vi "poly_control_signalling_write_caller_multi_2.vi"(6 "modes (Sgnl)":T1(array[ring]), 8 "error in (no error)":errorcluster, 9 "values":variant[](array[variant]), 10 "control names":string[](array[string]), 11 "name of caller in (your caller)":string) -> (0 "error out":errorcluster, 2 "control refs":refnum<vi>[](array[refnum]), 4 "found?":bool[](array[boolean]))   [LabVIEW 2015]
uses:
  poly_ref_tools_eco_plus.vi
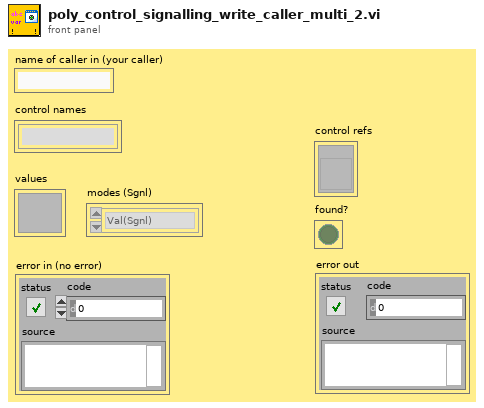
[diagram p1: front panel]
types:
  T1 = enum16{"Val", "Val(Sgnl)", "Val(Undo)", "Method"}[]
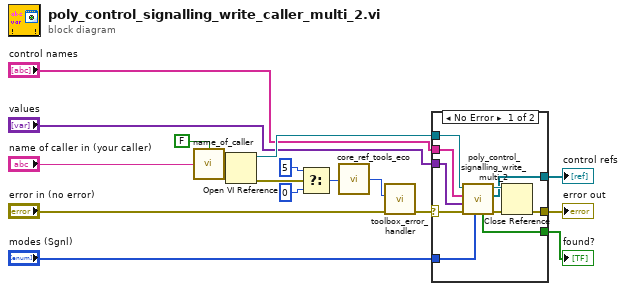
[diagram p0: block diagram]
diagram:
  n1 = call "name_of_caller.vi"("is in inlined vi? (F)"=FALSE, "name of caller in"="name of caller in (your caller)") -> ("name of caller out"=w16:string)  [unwired: 2 in]
  n2 = Open VI Reference(vi path=w16) -> (vi reference=w15:refnum<vi>, error out=w2:errorcluster)  [unwired: 5 in]
  n3 = Select(t=5, s=w2, f=0) -> (s? t:f=w5:i32)
  n4 = call-poly "core_ref_tools_eco.vi"("code (w/out eco)"=w5) -> ("code (+ eco)"=w4:i32)  [unwired: 4 in]
  n5 = call "toolbox_error_handler.vi"("error in (no error)"="error in (no error)", "code (0 = no error)"=w4) -> ("error out"=w1:errorcluster)  [unwired: 8 in, 1 out]
  n6 = case shown="No Error" w1 {
    selector: w1 -> [w18 w28]
    tunnel: w15 -> [w27 _]
    tunnel: [w24 w28] -> w14
    tunnel: [w23 _] -> w13
    tunnel: [w22 _] -> w12
    tunnel: "modes (Sgnl)" -> [w21 _]
    tunnel: "control names" -> [w20 _]
    tunnel: "values" -> [w19 _]
    frame No Error {
      n7 = call "poly_control_signalling_write_multi_2.vi"("modes (Sgnl)"=w21, "error in (no error)"=w18, "values"=w19, "control names"=w20, "vi reference"=w27) -> ("error out"=w25:errorcluster, "control refs"=w23:refnum<vi>[], "vi reference out"=w26:refnum<vi>, "found?"=w22:bool[])  [unwired: 3 in]
      n8 = Close Reference(reference=w26, error in (no error)=w25) -> (error out=w24:errorcluster)
    }
    frame Error {
    }
  }
  "error out" <- w14
  "found?" <- w12
  "control refs" <- w13
